vi "user login.vi"() -> ()   [LabVIEW 2019]
panel:
  out "Front Panel Window:Behavior":T1(ring)
  out "error out":errorcluster
  out "Username 2":refnum<vi>
  in  "Cancel":bool
  in  "OK":bool
  in  "Password":string
  in  "Username":string
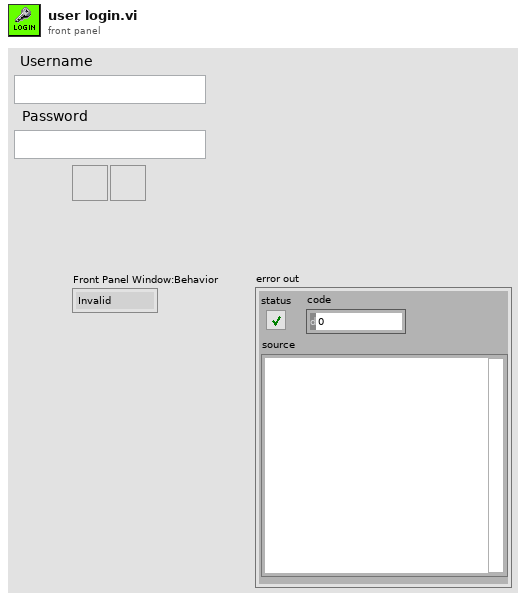
[diagram p1: front panel]
types:
  T1 = enum32{"Invalid", "Default", "Floating", "Floating/Auto-Hide", "Modal"}
  T2 = typedef "eventvkey.ctl" = enum16{"ASCII", "Enter", "Return", "Shift", "Ctrl", "Alt", "Cmd", "Opt", "Caps", "NumLock", "Clear", "Break", "Up", "Down", "Left", "Right", "Insert", "Delete", "Home", "End", "PageUp", "PageDown", "Escape", "Help", "Pause", "ScrollLock", "F1", "F2", "F3", "F4", "F5", "F6", "F7", "F8", "F9", "F10", "F11", "F12", "F13", "F14", "F15", "F16", "F17", "F18", "F19", "F20", "F21", "F22", "F23", "F24", "Play", "VolumeUp", "VolumeDown", "Mute", "Two Byte Char"}
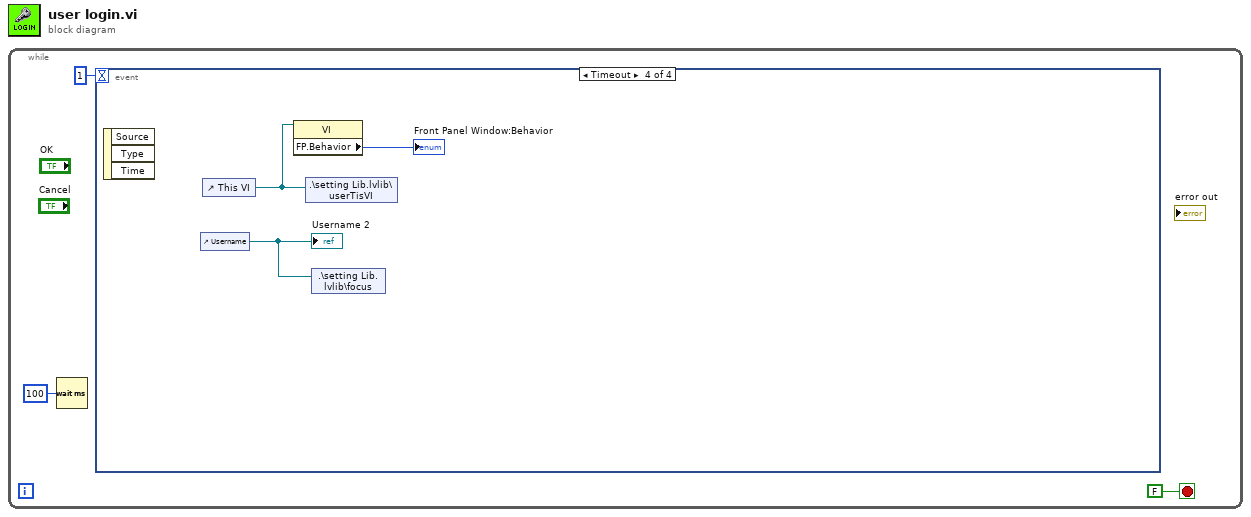
[diagram p0: block diagram]
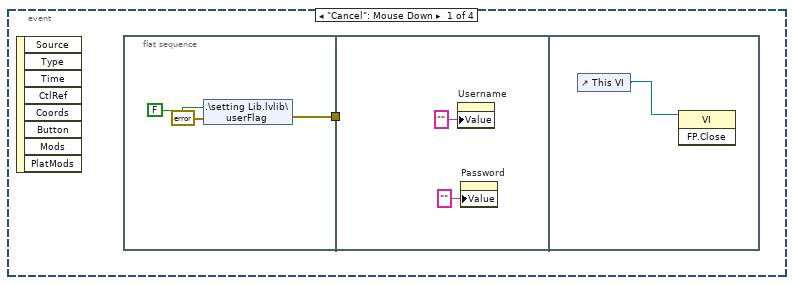
[diagram p2: hidden frame]
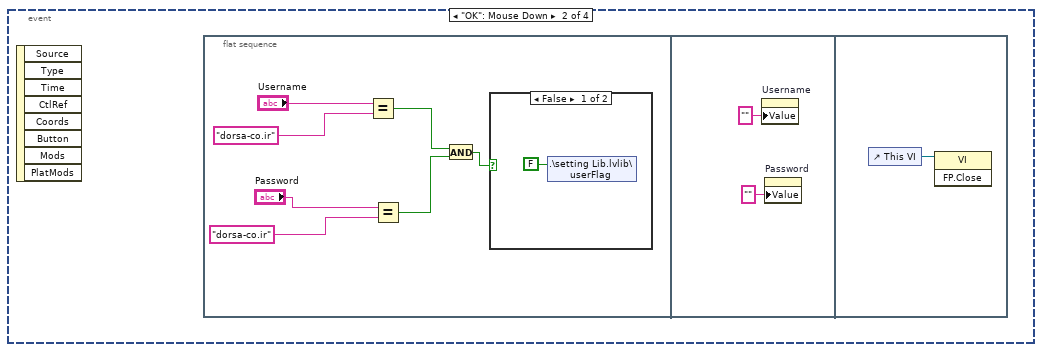
[diagram p3: hidden frame]
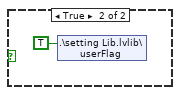
[diagram p4: hidden frame]
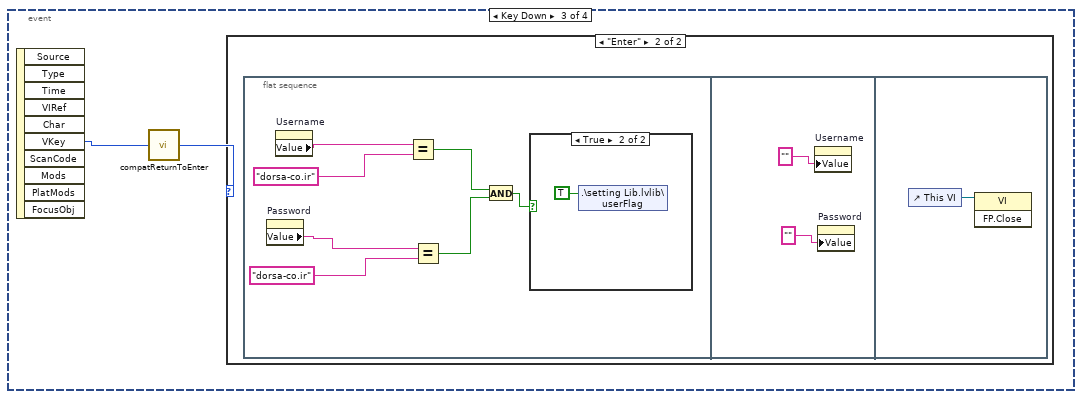
[diagram p5: hidden frame]
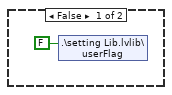
[diagram p7: hidden frame]
diagram:
  n1 = while {
    stop <- FALSE stop-if-true
    n2 = Wait (ms)(milliseconds to wait=u32 100) -> ()  [unwired: 1 out]
    n3 = event shown="[3] Timeout" {
      selector: _ -> [_ _ _ _]
      dyn-events: _ -> [_ _ _ _]
      timeout: 1 -> [_ _ _ _]
      event "Cancel": Mouse Down {
        n4 = event-data() -> ()  [unwired: 1 in, 8 out]
        n5 = flat-sequence {
          tunnel: [w6] -> w4
          tunnel: w4 -> [_]
          frame #0 {
            n6 = shared-variable ".\\setting Lib.lvlib\\userFlag"(FALSE ("userFlag"), error in=errorcluster {"status"=FALSE, "code"=0, "source"=""} ("error in (no error)")) -> (error out=w6:errorcluster)
          }
          frame #1 {
            n7 = property on="Username" class="Str"("Value"="" ("Username")) -> ()  [unwired: 2 in, 2 out]
            n8 = property on="Password" class="Str"("Value"="" ("Password")) -> ()  [unwired: 2 in, 2 out]
          }
          frame #2 {
            n9 = control-ref of="This VI"() -> (w10:refnum<vi>)
            n10 = invoke class="VI" method="FP.Close"(reference=w10) -> ()  [unwired: 2 in, 3 out]
          }
        }
      }
      event "OK": Mouse Down {
        n11 = event-data() -> ()  [unwired: 1 in, 8 out]
        n12 = flat-sequence {
          frame #0 {
            n13 = Equal?(x="Username", y="dorsa-co.ir") -> (x = y?=w13:bool)
            n14 = Equal?(x="Password", y="dorsa-co.ir") -> (x = y?=w12:bool)
            n15 = And(x=w13, y=w12) -> (x .and. y?=w11:bool)
            n16 = case shown="False" w11 {
              frame False {
                n17 = shared-variable ".\\setting Lib.lvlib\\userFlag"(FALSE ("userFlag")) -> ()  [unwired: 1 in, 1 out]
              }
              frame True {
                n18 = shared-variable ".\\setting Lib.lvlib\\userFlag"(TRUE ("userFlag")) -> ()  [unwired: 1 in, 1 out]
              }
            }
          }
          frame #1 {
            n19 = property on="Username" class="Str"("Value"="" ("Username")) -> ()  [unwired: 2 in, 2 out]
            n20 = property on="Password" class="Str"("Value"="" ("Password")) -> ()  [unwired: 2 in, 2 out]
          }
          frame #2 {
            n21 = control-ref of="This VI"() -> (w22:refnum<vi>)
            n22 = invoke class="VI" method="FP.Close"(reference=w22) -> ()  [unwired: 2 in, 3 out]
          }
        }
      }
      event Key Down {
        n23 = event-data() -> ("VKey"=w24:T2)  [unwired: 1 in, 9 out]
        n24 = call <vilib>:"compatReturnToEnter.vi"("VKey"=w24) -> ("VKey"=w23:T2)
        n25 = case shown="\"Enter\"" w23 {
          frame "ASCII", Default {
          }
          frame "Enter" {
            n26 = flat-sequence {
              frame #0 {
                n27 = property on="Password" class="Str"() -> ("Value"=w25:string)  [unwired: 2 in, 2 out]
                n28 = property on="Username" class="Str"() -> ("Value"=w26:string)  [unwired: 2 in, 2 out]
                n29 = Equal?(x=w26, y="dorsa-co.ir") -> (x = y?=w29:bool)
                n30 = Equal?(x=w25, y="dorsa-co.ir") -> (x = y?=w28:bool)
                n31 = And(x=w29, y=w28) -> (x .and. y?=w27:bool)
                n32 = case shown="True" w27 {
                  frame False {
                    n33 = shared-variable ".\\setting Lib.lvlib\\userFlag"(FALSE ("userFlag")) -> ()  [unwired: 1 in, 1 out]
                  }
                  frame True {
                    n34 = shared-variable ".\\setting Lib.lvlib\\userFlag"(TRUE ("userFlag")) -> ()  [unwired: 1 in, 1 out]
                  }
                }
              }
              frame #1 {
                n35 = property on="Username" class="Str"("Value"="" ("Username")) -> ()  [unwired: 2 in, 2 out]
                n36 = property on="Password" class="Str"("Value"="" ("Password")) -> ()  [unwired: 2 in, 2 out]
              }
              frame #2 {
                n37 = control-ref of="This VI"() -> (w36:refnum<vi>)
                n38 = invoke class="VI" method="FP.Close"(reference=w36) -> ()  [unwired: 2 in, 3 out]
              }
            }
          }
        }
      }
      event Timeout {
        n39 = event-data() -> ()  [unwired: 1 in, 3 out]
        n40 = control-ref of="Username"() -> (w39:refnum<vi>)
        "Username 2" <- w39
        n41 = control-ref of="This VI"() -> (w38:refnum<vi>)
        n42 = property class="VI"(reference=w38) -> ("FP.Behavior"=→"Front Panel Window:Behavior":T1)  [unwired: 1 in, 2 out]
        n43 = shared-variable ".\\setting Lib.lvlib\\userTisVI"(w38) -> ()  [unwired: 1 in, 1 out]
        n44 = shared-variable ".\\setting Lib.lvlib\\focus"(w39) -> ()  [unwired: 1 in, 1 out]
      }
    }
  }
